vi "WSVCAP SHL Host LL Calculate Wait Ticks.vi"(9 "Clock Rate (Hz)":dbl=50000.0, 13 "Simulate FPGA":bool) -> (4 "Wait Ticks":u32, 6 "Actual Rate (Hz)":dbl)   [LabVIEW 2017]
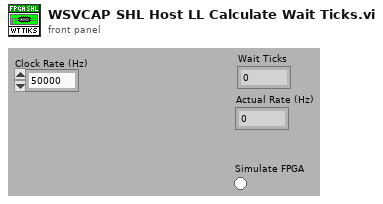
[diagram p1: front panel]
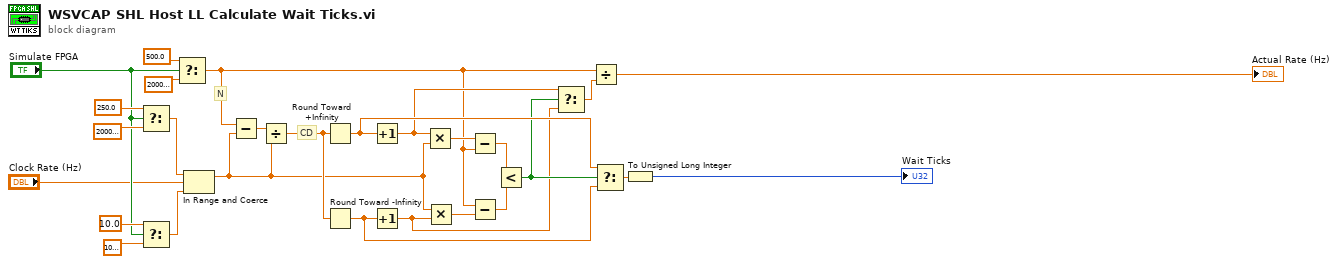
[diagram p0: block diagram]
diagram:
  # "CD"
  # "N"
  n1 = Select(t=250.0 ("10M"), s="Simulate FPGA", f=20000000.0 ("10M")) -> (s? t:f=w8:dbl)
  n2 = Select(t=10.0 ("10M"), s="Simulate FPGA", f=1000.0 ("10M")) -> (s? t:f=w4:dbl)
  n3 = Select(t=500.0 ("10M"), s="Simulate FPGA", f=20000000.0 ("10M")) -> (s? t:f=w13:dbl)
  n4 = In Range and Coerce(upper limit=w8, x="Clock Rate (Hz)", lower limit=w4) -> (coerced(x)=w3:dbl)  [unwired: 1 out]
  n5 = Subtract(x=w13, y=w3) -> (x-y=w23:dbl)
  n6 = Divide(x=w23, y=w3) -> (x/y=w22:dbl)
  n7 = Round Toward +Infinity(x=w22) -> (ceil(x): smallest int >= x=w21:dbl)
  n8 = Round Toward -Infinity(1:w22) -> (0:w20:dbl)
  n9 = Increment(x=w21) -> (x+1=w16:dbl)
  n10 = Increment(x=w20) -> (x+1=w17:dbl)
  n11 = Multiply(x=w16, y=w3) -> (x*y=w27:dbl)
  n12 = Multiply(x=w3, y=w17) -> (x*y=w26:dbl)
  n13 = Subtract(x=w27, y=w13) -> (x-y=w24:dbl)
  n14 = Subtract(x=w13, y=w26) -> (x-y=w25:dbl)
  n15 = Less?(x=w24, y=w25) -> (x < y?=w18:bool)
  n16 = Select(t=w16, s=w18, f=w17) -> (s? t:f=w19:dbl)
  n17 = Divide(x=w13, y=w19) -> (x/y=→"Actual Rate (Hz)":dbl)
  n18 = Select(t=w21, s=w18, f=w20) -> (s? t:f=w12:dbl)
  n19 = To Unsigned Long Integer(number=w12) -> (unsigned 32bit integer=→"Wait Ticks":u32)
